vi "HAL camera quit.vi"() -> ()   [LabVIEW 2011]
uses:
  Cascade-specific globals.vi
panel:
  out "error out":errorcluster
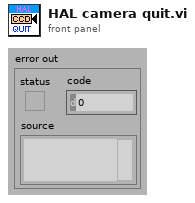
[diagram p1: front panel]
types:
  T1 = cluster{"Camera Handle":u32, "Pulser Handle":u32, "File Handle":u32, "Display Handle":u32, "Image Handle":u32}
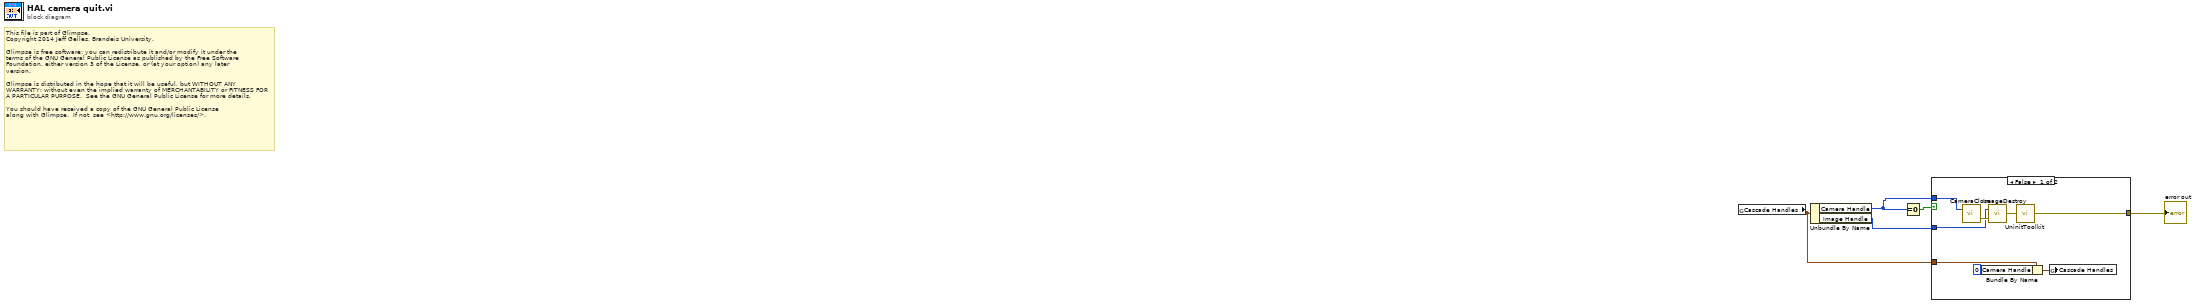
[diagram p0: block diagram]
diagram:
  # "This file is part of Glimpse. \nCopyright 2014 Jeff Gelles, Brandeis University.    \n\nGlimpse is free software: you can redistribute it and/or modify it under the \nterms of the GNU General Public License as published by the Free Software \nFoundation, either version 3 of the License, or (at your option) any later \nversion.\n\nGlimpse is distributed in the hope that it will be useful, but WITHOUT ANY \nWARRANTY; without even the implied warranty of MERCHANTABILITY or FITNESS FOR \nA PARTICULAR PURPOSE.  See the GNU General Public License for more details.\n\nYou should have received a copy of the GNU General Public License\nalong with Glimpse.  If not, see <http://www.gnu.org/licenses/>."
  n1 = global read "Cascade-specific globals.vi" "Cascade Handles"() -> (w1:T1)
  n2 = Unbundle By Name(w1) -> ("Camera Handle"=w3:u32, "Image Handle"=w2:u32)
  n3 = Equal To 0?(x=w3) -> (x = 0?=w4:bool)
  n4 = case shown="False" w4 {
    tunnel: w3 -> [w11 _]
    tunnel: w2 -> [w10 _]
    tunnel: [w9 _] -> w5
    tunnel: w1 -> [w8 _]
    frame False {
      n5 = call <userlib>:"CameraClose.vi"("Camera Handle"=w11) -> ("error out"=w12:errorcluster)  [unwired: 1 in]
      n6 = Bundle By Name(cluster=w8, "Camera Handle"=u32 0) -> (w7:T1)
      n7 = call <userlib>:"ImageDestroy.vi"("error in"=w12, "Data handle"=w10) -> ("error out"=w13:errorcluster)
      n8 = call <userlib>:"UninitToolkit.vi"("error in"=w13) -> ("error out"=w9:errorcluster)
      n9 = global write "Cascade-specific globals.vi" "Cascade Handles"(w7) -> ()
    }
    frame True {
    }
  }
  "error out" <- w5
